vi "Assert Is Boolean.vi"(7 "Message (\"\")":string, 8 "error in (no error)":errorcluster, 10 "Actual":variant) -> (0 "error out":errorcluster)   [LabVIEW 2017, in "Transparent Assertions.lvlib" / "Assertions.lvlib"]
doc: "Asserts that a variable is of Boolean type."
uses:
  Assertions.lvlib
  <vilib>/Utility/Data Type/Type Definitions/Data Type.ctl
  Constraints/IsType/IsType.lvclass
  <vilib>/Utility/Data Type/NI_Data Type.lvlib
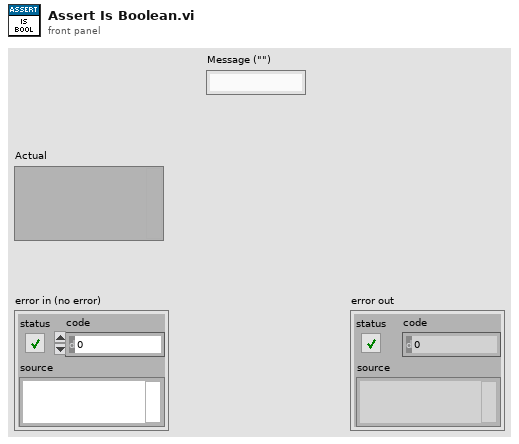
[diagram p1: front panel]
types:
  T1 = typedef "NI_Data Type.lvlib/Data Type.ctl" = enum8{"Invalid Type", "Void", "I8", "I16", "I32", "I64", "U8", "U16", "U32", "U64", "Single Float", "Double Float", "Extended Float", "Single Complex", "Double Complex", "Extended Complex", "Enum U8", "Enum U16", "Enum U32", "Enum U64", "Single Float With Unit", "Double Float With Unit", "Extended Float With Unit", "Single Complex with Unit", "Double Complex with Unit", "Extended Complex with Unit", "Boolean", "String", "Path", "Picture", "Tag", "Array", "Cluster", "Variant", "LV Variant", "Waveform", "Timestamp", "Digital Waveform", "Digital Data", "ExpressData", "Refnum", "External Data", "VI", "Poly VI", "LabVIEW Class Instance", "Fixed Point"}
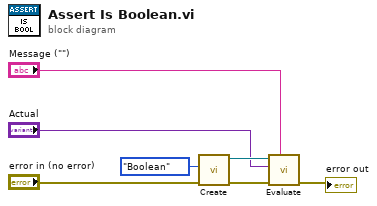
[diagram p0: block diagram]
diagram:
  n1 = call "Create.vi"("error in (no error)"="error in (no error)", "Expected"=Data_Type."Boolean") -> ("error out"=w6:errorcluster, "IsType"=w3:refnum<class "IsType.lvclass">)  [unwired: 8 in]
  n2 = call-dynamic "Evaluate.vi"("Message (\"\")"="Message (\"\")", "error in (no error)"=w6, "Actual"="Actual", "Constraint in"=w3) -> ("error out"=→"error out":errorcluster)  [unwired: 6 in, 1 out]
